vi "main.vi"() -> ()   [LabVIEW 2020]
uses:
  <vilib>/Instr/_visa.llb/VISA Configure Serial Port (Instr).vi
panel:
  in  "Stopp":bool
  in  "?":u16 max=1000
  out "?":i32(graph)
  out "?":bool
  in  "Controller":string="Arduino"
  in  "write":bool
  in  "Baud Rate":u32=9600
  out "?":string
  in  "stop":bool
  # "Smart Pump Control Panel"
  # "Arduino Connection"
  # "Sensor Value [mBar]"
  # "Set Pressure [mBar]"
  # "Sensor Value [mBar]"
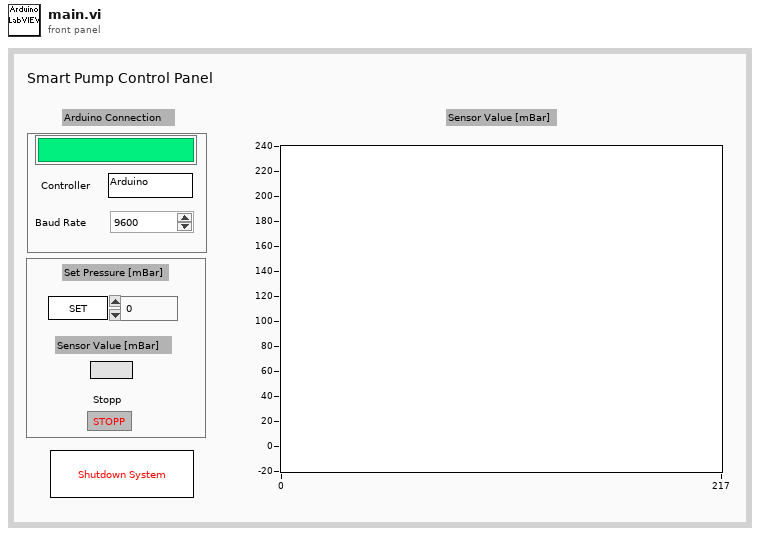
[diagram p1: front panel]
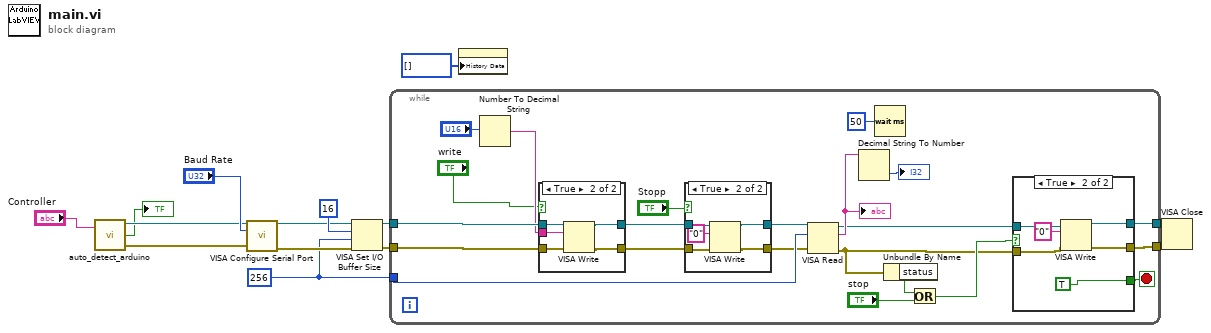
[diagram p0: block diagram]
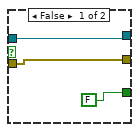
[diagram p3: hidden frame]
diagram:
  w1 = u32 256 ("buffer size")
  n1 = call "auto_detect_arduino.vi"("instr name"="Controller") -> ("VISA resource name"=w11:refnum<visa-resource-name>, "status"=→"?":bool, "error out"=w10:errorcluster)  [unwired: 1 in]
  n2 = call-poly "VISA Configure Serial Port"("VISA resource name"=w11, "baud rate (9600)"="Baud Rate", "error in (no error)"=w10) -> ("VISA resource name out"=w7:refnum<visa-resource-name>, "error out"=w6:errorcluster)  [unwired: 11 in]
  n3 = VISA Set I/O Buffer Size(VISA resource name=w7, mask (16)=u16 16 ("I/O Receive\nBuffer mask"), size (4096)=w1, error in (no error)=w6) -> (VISA resource name out=w5:refnum<visa-resource-name>, error out=w4:errorcluster)
  n4 = while {
    tunnel: w5 -> [w33]
    tunnel: w4 -> [w32]
    tunnel: [w24] -> w14
    tunnel: [w23] -> w13
    tunnel: w1 -> [w34]
    stop <- w21 stop-if-true
    n5 = Number To Decimal String(number="?") -> (decimal integer string=w27:string)  [unwired: 1 in]
    n6 = case shown="True" "write" {
      tunnel: w33 -> [w54 w59]
      tunnel: w32 -> [w53 w58]
      tunnel: [w54 w57] -> w19
      tunnel: [w53 w56] -> w18
      tunnel: w27 -> [_ w55]
      frame False {
      }
      frame True {
        n7 = VISA Write(VISA resource name=w59, write buffer=w55, error in (no error)=w58) -> (VISA resource name out=w57:refnum<visa-resource-name>, error out=w56:errorcluster)  [unwired: 1 out]
      }
    }
    n8 = case shown="True" "Stopp" {
      tunnel: w19 -> [w38 w40]
      tunnel: w18 -> [w37 w41]
      tunnel: [w38 w43] -> w17
      tunnel: [w37 w42] -> w16
      frame False {
      }
      frame True {
        n9 = VISA Write(VISA resource name=w40, write buffer="0" ("Schreibpuffer"), error in (no error)=w41) -> (VISA resource name out=w43:refnum<visa-resource-name>, error out=w42:errorcluster)  [unwired: 1 out]
      }
    }
    n10 = VISA Read(VISA resource name=w17, byte count=w34, error in (no error)=w16) -> (VISA resource name out=w25:refnum<visa-resource-name>, read buffer=w30:string, error out=w22:errorcluster)  [unwired: 1 out]
    "?" <- w30
    n11 = Decimal String To Number(string=w30) -> (number=→"?":i32)  [unwired: 2 in, 1 out]
    n12 = Wait (ms)(milliseconds to wait=u32 50) -> ()  [unwired: 1 out]
    n13 = Unbundle By Name(w22) -> ("status"=w36:bool)
    n14 = Or(x=w36, y="stop") -> (x .or. y?=w26:bool)
    n15 = case shown="True" w26 {
      tunnel: w25 -> [w46 w52]
      tunnel: [w46 w51] -> w24
      tunnel: [w45 w50] -> w23
      tunnel: w22 -> [w45 w49]
      tunnel: [FALSE TRUE] -> w21
      frame False {
      }
      frame True {
        n16 = VISA Write(VISA resource name=w52, write buffer="0" ("Schreibpuffer"), error in (no error)=w49) -> (VISA resource name out=w51:refnum<visa-resource-name>, error out=w50:errorcluster)  [unwired: 1 out]
      }
    }
  }
  n17 = property class="SVDiagr (strikt)"("History Data"=i32[] []) -> ()  [unwired: 2 in, 2 out]
  n18 = VISA Close(VISA resource name=w14, error in (no error)=w13) -> ()  [unwired: 1 out]
